vi "RDB Create Objects Receive.vi"(8 "error in (no error)":errorcluster, 11 "RDB Data Receive":T4) -> (0 "error out":errorcluster, 3 "RDB Reference":T1 {"RDB Data"."payload" format="%x"; "RDB Data"."timestamp" format="%<%.7X\n%x>T"; "RDB Data"."type" items=["FlexRay Data"=32, "FlexRay Null"=33, "FlexRay Symbol"=34, "Log Trigger"=225, "Start Trigger"=226]; "RDB Data"."cycle count" max=63 step=1})   [LabVIEW 2023, in "RDB.lvlib"]
uses:
  RDB.lvlib
  System Explorer/RDB Data.ctl
  RDB Object.ctl
  RDB Player Object.ctl
  RDB Reference.ctl
  <vilib>/xnet/xnet.llb/XNET Frame FlexRay.ctl
  <vilib>/xnet/xnet.llb/XNET Frame Type FlexRay.ctl
  <vilib>/xnet/xnet.llb/XNET String To IO Name (Signal).vi
  <vilib>/xnet/xnet.llb/XNET Create Session (Conversion).vi
  <resource>/objmgr/xnet.rc
  Shared/Vires VTD Shared.lvlib
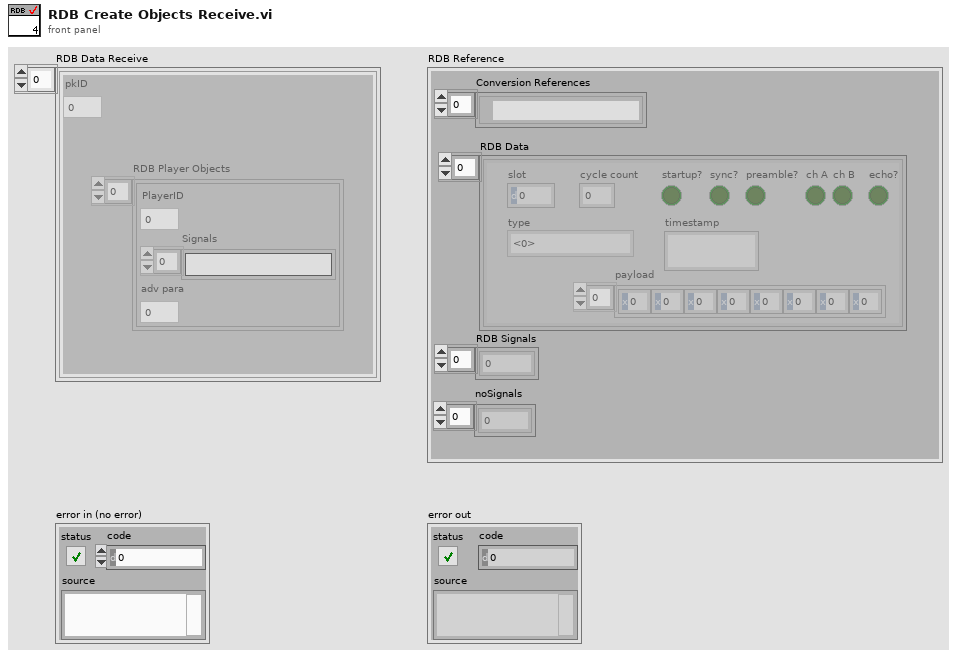
[diagram p1: front panel]
types:
  T1 = typedef "RDB.lvlib/RDB Reference.ctl" = cluster{"Conversion References":refnum<k21>[], "RDB Data":T2[], "RDB Signals":dbl[], "noSignals":i32[]}
  T2 = typedef "XNET Frame FlexRay.ctl" = cluster{"timestamp":timestamp, "payload":u8[], "slot":u16, "type":T3, "cycle count":u8, "startup?":bool, "sync?":bool, "preamble?":bool, "ch A":bool, "ch B":bool, "echo?":bool}
  T3 = typedef "XNET Frame Type FlexRay.ctl" = u8
  T4 = typedef "Vires VTD Shared.lvlib/RDB Data.ctl" = T5[]
  T5 = typedef "RDB.lvlib/RDB Object.ctl" = cluster{"pkID":i32, "RDB Player Objects":T6[]}
  T6 = typedef "RDB.lvlib/RDB Player Object.ctl" = cluster{"PlayerID":i32, "Signals":string[], "adv para":i32}
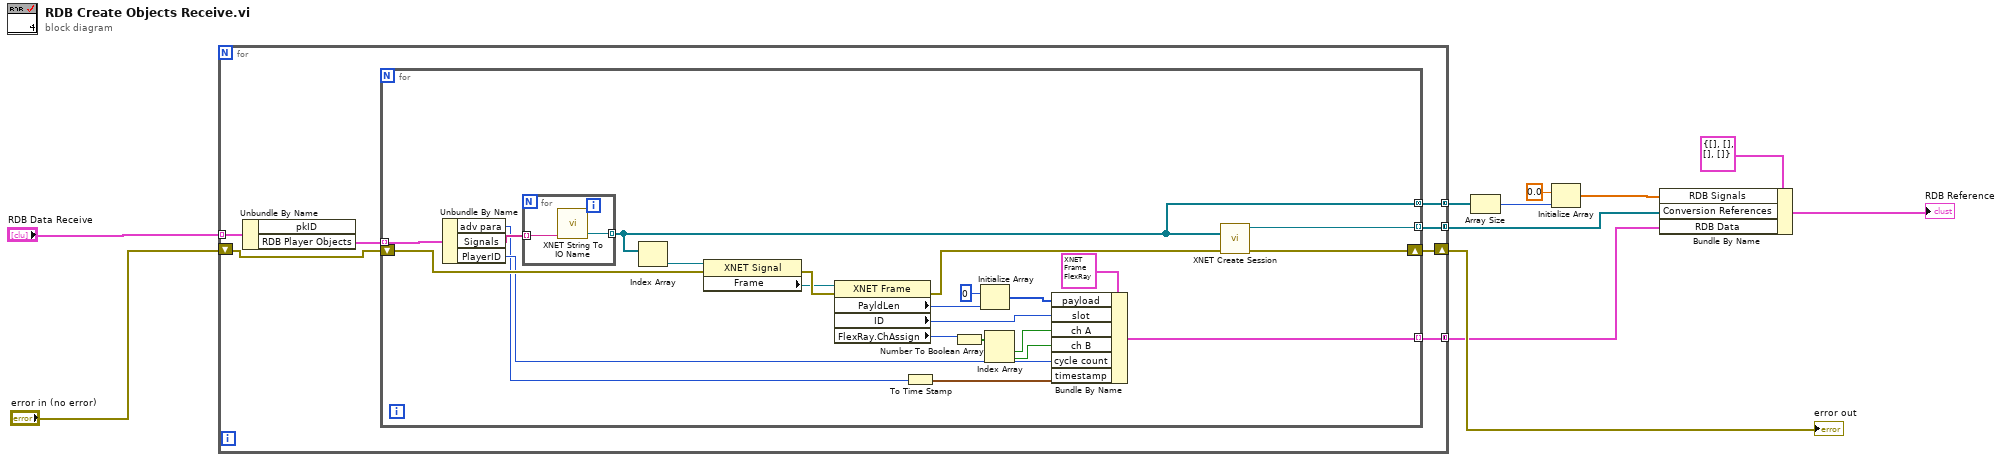
[diagram p0: block diagram]
diagram:
  n1 = for {
    tunnel: "RDB Data Receive" -> [w18] mode=indexing
    shift-right: [w16] -> w11
    shift-left: "error in (no error)" -> [w15]
    tunnel: [w14] -> w4 mode=concatenating
    tunnel: [w12] -> w5 mode=concatenating
    tunnel: [w13] -> w6 mode=concatenating
    n2 = Unbundle By Name(w18) -> ("RDB Player Objects"=w17:T6[])  [unwired: 1 out]
    n3 = for {
      tunnel: w17 -> [w41] mode=indexing
      shift-right: [w40] -> w16
      shift-left: w15 -> [w39]
      tunnel: [w38] -> w14 mode=concatenating
      tunnel: [w23] -> w13 mode=indexing
      tunnel: [w19] -> w12 mode=indexing
      n4 = Unbundle By Name(w41) -> ("adv para"=w21:i32, "Signals"=w36:string[], "PlayerID"=w24:i32)
      n5 = for {
        tunnel: w36 -> [w42] mode=indexing
        tunnel: [w43] -> w38 mode=indexing
        n6 = call-poly <vilib>:"XNET String To IO Name.vi"("string"=w42) -> ("XNET Signal"=w43:refnum<k21>)  [unwired: 4 out]
      }
      n7 = Index Array(array=w38) -> (element=w25:refnum<k21>)  [unwired: 1 in]
      n8 = property class="XNET Signal"(reference=w25, error in=w39) -> (error out=w35:errorcluster, "Frame"=w34:refnum<k21>)  [unwired: 1 out]
      n9 = property class="XNET Frame"(reference=w34, error in=w35) -> (error out=w37:errorcluster, "PayldLen"=w27:u32, "ID"=w29:u32, "FlexRay.ChAssign"=w30:u32)  [unwired: 1 out]
      n10 = To Time Stamp(1:w21) -> (0:w20:timestamp)
      n11 = Number To Boolean Array(number=w30) -> (Boolean array=w26:bool[])
      n12 = Initialize Array(0 ("element"), w27) -> (w28:i32[])
      n13 = Index Array(array=w26) -> (element #1=w31:bool, element #2=w32:bool)  [unwired: 2 in]
      n14 = Bundle By Name(cluster=T2 {"timestamp"=timestamp(0 s since 1904-01-01), "payload"=[], "slot"=1, "type"=32, "cycle count"=0, "startup?"=FALSE, "sync?"=FALSE, "preamble?"=FALSE, "ch A"=FALSE, "ch B"=FALSE, "echo?"=FALSE} ("FlexRay frame"), "payload"=w28, "slot"=w29, "ch A"=w31, "ch B"=w32, "cycle count"=w24, "timestamp"=w20) -> (w23:T2)
      n15 = call-poly <vilib>:"XNET Create Session.vi"("signal list"=w38, "error in (no error)"=w37) -> ("session out"=w19:refnum<k21>, "error out"=w40:errorcluster)  [unwired: 12 in]
    }
  }
  "error out" <- w11
  n16 = Array Size(array=w4) -> (size(s)=w3:i32)
  n17 = Initialize Array(0.0 ("element"), w3) -> (w2:dbl[])
  n18 = Bundle By Name(cluster=T1 {"Conversion References"=[], "RDB Data"=[], "RDB Signals"=[], "noSignals"=[]} ("RDB Reference"), "RDB Signals"=w2, "Conversion References"=w5, "RDB Data"=w6) -> (→"RDB Reference":T1)
